vi "Write Micron Optics Digitizer Configuration.vi"(8 "error in (no error)":errorcluster, 10 "Micron Optics Digitizer Configuration":T1={"Post-trigger delay"=0.01, "Post-trigger duration"=0.1, "Rate"=1000000.0, "Reference channel"=-1, "Detection Setting IDs"=[130, 130], "Stream and average"=FALSE, "Address"="10.0.0.55"} {"Rate" format="%#_8pHz"; "Post-trigger duration" format="%#_6ps"; "Post-trigger delay" format="%#_6ps"}, 11 "Micron Optics Driver in":refnum<class "Micron Optics Driver.lvclass">) -> (0 "error out":errorcluster, 3 "Micron Optics Driver out":refnum<class "Micron Optics Driver.lvclass">)   [LabVIEW 2024, in "Micron Optics Driver.lvclass"]
uses:
  Micron Optics Driver.lvclass
  Micron optics didgitizer configuration.ctl
  Micron Optics Driver.lvclass/Micron Optics Driver.ctl
panel:
  # "Pulse config"
  # "Monitor config"
  # "CH1\n.\n.\n.\n.\n.\nCH4"
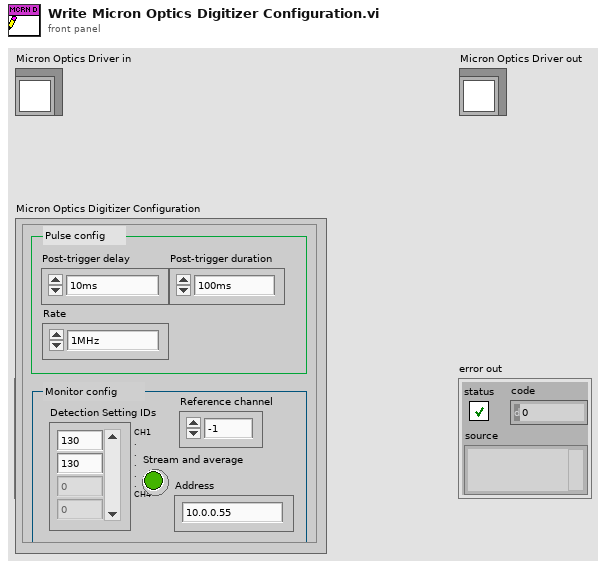
[diagram p1: front panel]
types:
  T1 = typedef "Micron optics didgitizer configuration.ctl" = cluster{"Post-trigger delay":dbl, "Post-trigger duration":dbl, "Rate":dbl, "Reference channel":i32, "Detection Setting IDs":u8[], "Stream and average":bool, "Address":string}
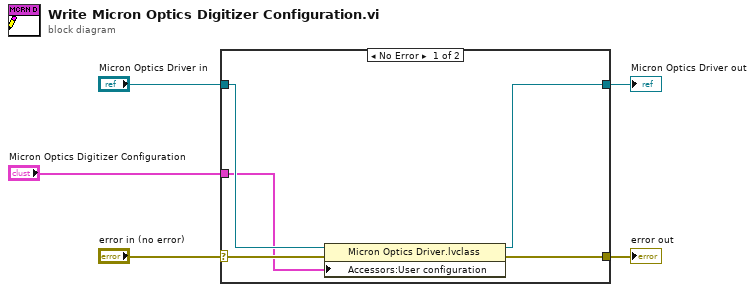
[diagram p0: block diagram]
diagram:
  n1 = case shown="No Error" "error in (no error)" {
    selector: "error in (no error)" -> [w10 w11]
    tunnel: [w9 w11] -> w4
    tunnel: [w7 w12] -> w2
    tunnel: "Micron Optics Driver in" -> [w8 w12]
    tunnel: "Micron Optics Digitizer Configuration" -> [w6 _]
    frame No Error {
      n2 = property class="Micron Optics Driver.lvclass"(reference=w8, error in=w10, "Accessors:User configuration"=w6) -> (reference out=w7:refnum<class "Micron Optics Driver.lvclass">, error out=w9:errorcluster)
    }
    frame Error {
    }
  }
  "error out" <- w4
  "Micron Optics Driver out" <- w2
